vi "_get_spec_list.vi"(8 "error in (no error)":errorcluster, 9 "RequiredSizeInput":u32, 10 "ListSizeInput":u32, 11 "UV-VIS_AVANTES in":refnum<class "UV-VIS_AVANTES.lvclass">) -> (0 "error out":errorcluster, 1 "List Output":u8[](array[numeric]), 3 "UV-VIS_AVANTES out":refnum<class "UV-VIS_AVANTES.lvclass">)   [LabVIEW 2020, in "UV-VIS_AVANTES.lvclass"]
uses:
  UV-VIS_AVANTES.lvclass
  C:/Dev/TRANCON/Classes/Detector/Detector.lvclass
  Detector.lvclass/Detector.ctl
  UV-VIS_AVANTES.lvclass/UV-VIS_AVANTES.ctl
  Detector.lvclass
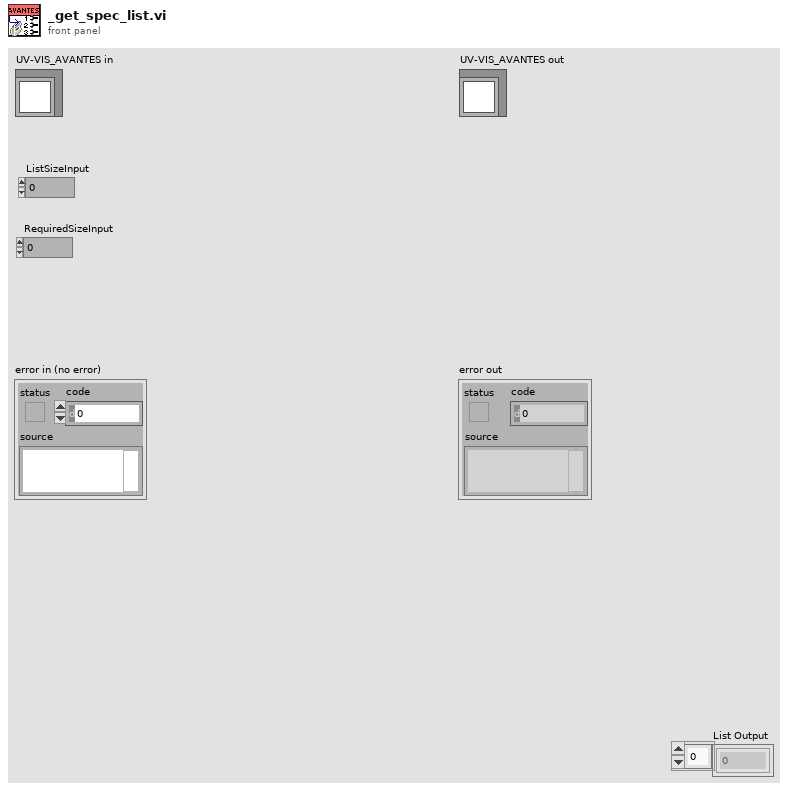
[diagram p1: front panel]
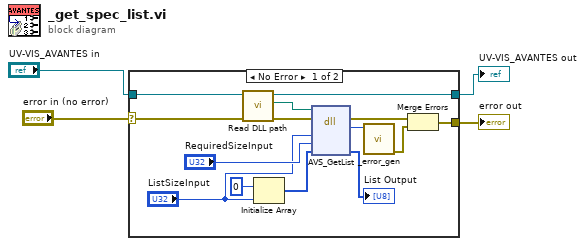
[diagram p0: block diagram]
diagram:
  n1 = case shown="No Error" "error in (no error)" {
    selector: "error in (no error)" -> [w17 w20]
    tunnel: [w5 w20] -> w3
    tunnel: [w16 w19] -> w1
    tunnel: "UV-VIS_AVANTES in" -> [w18 w19]
    frame No Error {
      n2 = call "Read DLL path.vi"("error in (no error)"=w17, "Detector in"=w18) -> ("error out"=w12:errorcluster, "DLL path"=w13:path, "Detector out"=w16:refnum<class "UV-VIS_AVANTES.lvclass">)  [unwired: 7 in]
      n3 = Initialize Array(u8 0, "ListSizeInput") -> (w9:u8[])
      n4 = dll-call lib="C:/AvaSpecX64-DLL_9.4/examples/LabView/LabViewSingleChan/avaspec.dll" fn="AVS_GetList"(path in=w13, error in=w12, "a_ListSize"="ListSizeInput", "a_pRequiredSize"="RequiredSizeInput", "a_pList"=w9) -> (error out=w7:errorcluster, "return type"=w6:i32, "a_pList"=→"List Output":u8[])  [unwired: 3 in, 1 out]
      n5 = call "_error_gen.vi"("return type"=w6) -> ("error out"=w8:errorcluster)  [unwired: 10 in]
      n6 = Merge Errors(w7, w8) -> (w5:errorcluster)
    }
    frame Error {
    }
  }
  "error out" <- w3
  "UV-VIS_AVANTES out" <- w1
